vi "医保刷卡记录系统.vi"() -> ()   [LabVIEW 2017]
uses:
  <vilib>/Platform/TimedLoop/XDataNode/timing_clust.ctl
  <vilib>/Platform/TimedLoop/XDataNode/nitl_modes.ctl
  <vilib>/Platform/TimedLoop/XDataNode/wakeup.ctl
  <vilib>/Platform/TimedLoop/XDataNode/XDataNode.xnode
  <vilib>/Platform/TimedLoop/XDataNode/XDNodeRunTimeDep.lvlib
panel:
  out "药费总额":dbl
  out "化验费总额":dbl
  out "诊疗费用总额":dbl
  out "一般材料总额":dbl
  in  "数据清空":bool
  out "数据条数":i32
  in  "数组":T1(array[cluster])
  in  "添加数据":bool
  in  "药费":dbl
  in  "化验费":dbl
  in  "诊疗费用":dbl
  in  "一般材料":dbl
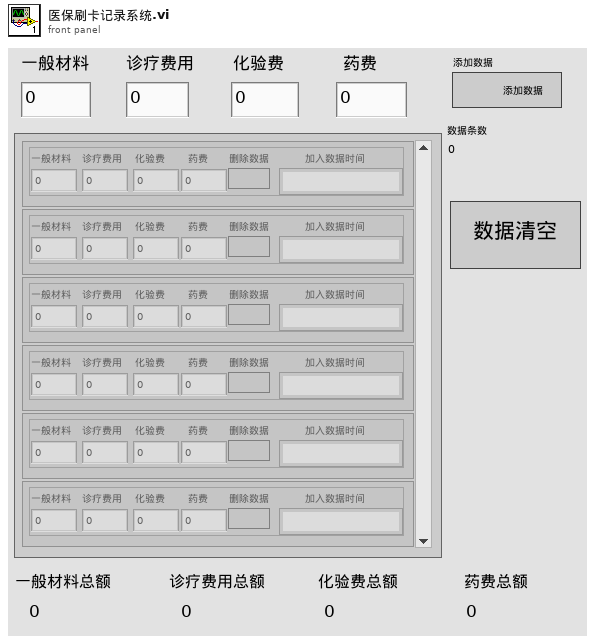
[diagram p1: front panel]
types:
  T1 = cluster{"一般材料":dbl, "诊疗费用":dbl, "化验费":dbl, "药费":dbl, "删除数据":bool, "加入数据时间":string}[]
  T2 = typedef "XDNodeRunTimeDep.lvlib/timing_clust.ctl" = cluster{"Expected End [f-1]":u64, "Actual End [f-1]":u64, "Finished Late? [f-1]":bool, "Expected End [i-1]":u64, "Actual End [i-1]":u64, "Finished Late? [i-1]":bool, "Expected Start [i]":u64, "Actual Start [i]":u64, "Expected Start [f]":u64, "Actual Start [f]":u64, "Source Name":string, "Structure Name":string, "Period":i64, "Deadline":i64, "Offset":i64, "Start":i64, "Priority":i32, "Timeout":i32, "Mode":T3, "Wakeup Reason":T4, "Error":errorcluster, "Source Type":string, "Secondary Source Type":string, "Global End Time":u64, "Global Start Time":u64, "Frame Duration":u64, "Iteration Duration":u64, "Assigned CPU":i32, "I/O Scan Engine Mode":u32}
  T3 = typedef "XDNodeRunTimeDep.lvlib/nitl_modes.ctl" = enum32{"No Change", "Process missed periods, maintain original phase", "Discard missed periods, maintain original phase", "Process missed periods, ignore original phase", "Discard missed periods, ignore original phase"}
  T4 = typedef "XDNodeRunTimeDep.lvlib/wakeup.ctl" = enum32{"Normal", "Aborted", "Asynchronous wakeup", "Timing source error", "Timed loop error", "Timeout"}
  T5 = cluster{"一般材料":dbl, "诊疗费用":dbl, "化验费":dbl, "药费":dbl, bool, string}[]
  T6 = cluster{"一般材料":dbl, "诊疗费用":dbl, "化验费":dbl, "药费":dbl, bool, string}
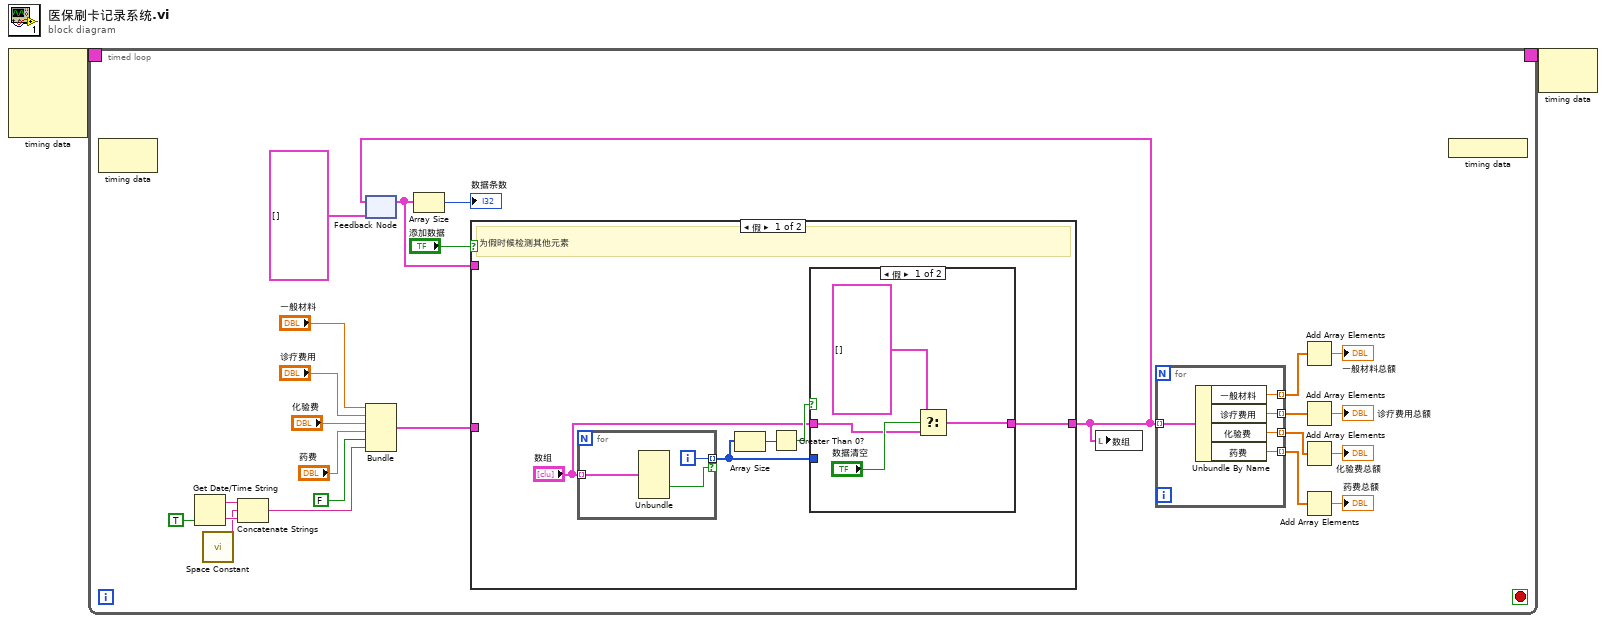
[diagram p0: block diagram]
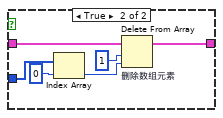
[diagram p2: hidden frame]
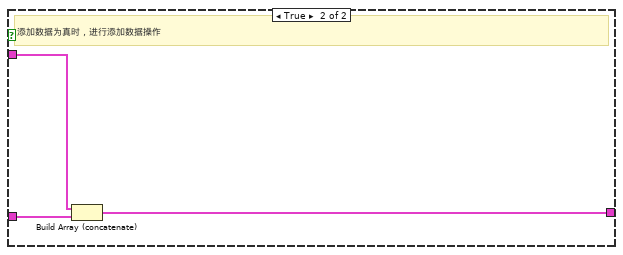
[diagram p3: hidden frame]
diagram:
  n1 = node-c288() -> (w2:T2)  [unwired: 4 in]
  n2 = timed-loop {
    timing: w2 -> [_]
    timing-out: [_] -> w1
    stop <- _ stop-if-true
    n3 = node-c288() -> ()  [unwired: 1 in, 1 out]
    n4 = Get Date/Time String(want seconds? (F)=TRUE ("需要秒？(F)")) -> (date string=w20:string, time string=w19:string)  [unwired: 2 in]
    n5 = call <vilib>:"Space Constant.vi"() -> ("String"=w18:string)
    n6 = Concatenate Strings(w20, w18, w19) -> (w17:string)
    n7 = feedback #1(T5 []) -> (w13:T5)
    n8 = Bundle("一般材料"="一般材料", "诊疗费用"="诊疗费用", "化验费"="化验费", "药费"="药费", FALSE, w17) -> (w16:T6)  [unwired: 1 in]
    n9 = Array Size(array=w13) -> (size(s)=→"数据条数":i32)
    n10 = case "条件结构" shown="假" "添加数据" {
      tunnel: w16 -> [_ w52]
      tunnel: [w33 w51] -> w11
      tunnel: w13 -> [_ w50]
      frame False {
        # "为假时候检测其他元素"
        n11 = for {
          tunnel: [w49] -> w36 mode=indexing if=w47
          tunnel: "数组" -> [w48] mode=indexing
          i -> [w49]
          n12 = Unbundle(w48) -> ("删除数据"=w47:bool)  [unwired: 5 out]
        }
        n13 = Array Size(array=w36) -> (size(s)=w35:i32)
        n14 = Greater Than 0?(x=w35) -> (x > 0?=w34:bool)
        n15 = case shown="假" w34 {
          tunnel: w36 -> [_ w46]
          tunnel: [w38 w42] -> w33
          tunnel: "数组" -> [w39 w41]
          frame False {
            n16 = Select(t=T1 [], s="数据清空", f=w39) -> (s? t:f=w38:T1)
          }
          frame True {
            n17 = Index Array(array=w46, index=0 ("索引")) -> (element=w45:i32)
            n18 = Delete From Array "删除数组元素"(array=w41, length=1 ("长度"), index=w45) -> (array with subset deleted=w42:T1)  [unwired: 1 out]
          }
        }
      }
      frame True {
        # "添加数据为真时，进行添加数据操作"
        n19 = Build Array (concatenate)(w50, w52) -> (w51:T5)
      }
    }
    n20 = feedback-in #1(w11) -> ()
    n21 = local write "数组"(w11) -> ()
    n22 = for {
      tunnel: w11 -> [w31] mode=indexing
      tunnel: [w30] -> w10 mode=indexing
      tunnel: [w29] -> w9 mode=indexing
      tunnel: [w28] -> w7 mode=indexing
      tunnel: [w27] -> w8 mode=indexing
      n23 = Unbundle By Name(w31) -> ("一般材料"=w30:dbl, "诊疗费用"=w29:dbl, "化验费"=w28:dbl, "药费"=w27:dbl)
    }
    n24 = Add Array Elements(numeric array=w10) -> (sum=→"一般材料总额":dbl)
    n25 = Add Array Elements(numeric array=w9) -> (sum=→"诊疗费用总额":dbl)
    n26 = Add Array Elements(numeric array=w7) -> (sum=→"化验费总额":dbl)
    n27 = Add Array Elements(numeric array=w8) -> (sum=→"药费总额":dbl)
    n28 = node-c288() -> ()  [unwired: 1 out]
  }
  n29 = node-c288(w1) -> ()  [unwired: 1 out]
